vi "Read an entire module using Varaible Nodes.vi"() -> ()   [LabVIEW 2025]
panel:
  in  "stop":bool
  out "Data":dbl[](array[numeric])
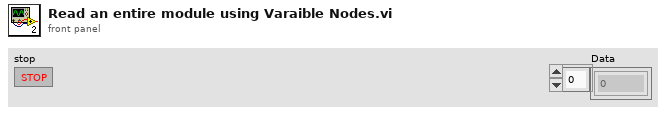
[diagram p1: front panel]
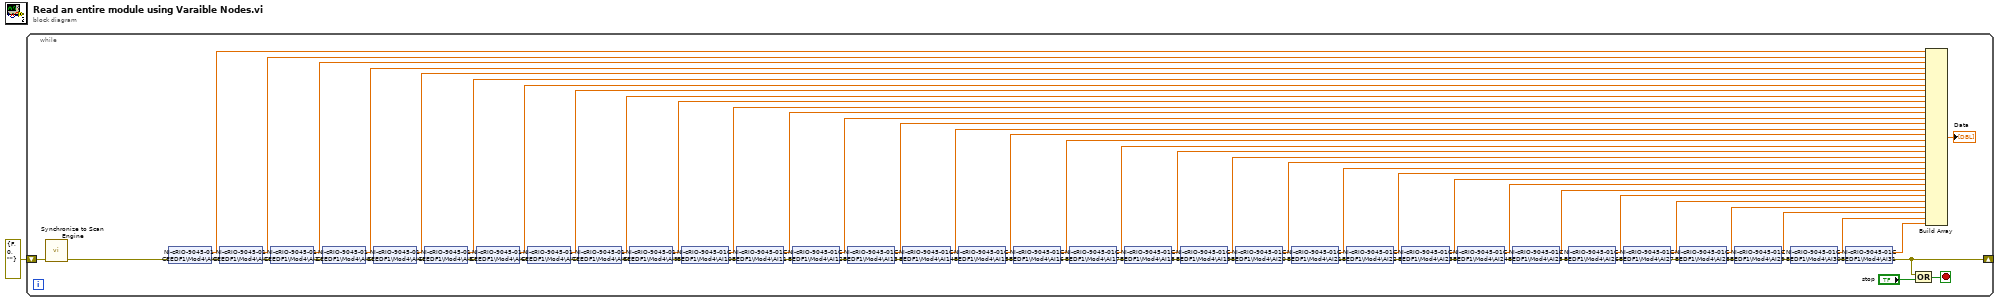
[diagram p0: block diagram]
diagram:
  n1 = while {
    shift-right: [w3] -> _
    shift-left: errorcluster {"status"=FALSE, "code"=0, "source"=""} ("error IO") -> [w2]
    stop <- w5 stop-if-true
    n2 = call <vilib>:"Synchronize to Scan Engine.vi"("error in (no error)"=w2) -> ("error out"=w4:errorcluster)  [unwired: 9 in, 1 out]
    n3 = shared-variable "NI-cRIO-9045-01CEEDF1\\Mod4\\AI0"(error in=w4) -> (w8:dbl, error out=w70:errorcluster)
    n4 = shared-variable "NI-cRIO-9045-01CEEDF1\\Mod4\\AI1"(error in=w70) -> (w9:dbl, error out=w69:errorcluster)
    n5 = shared-variable "NI-cRIO-9045-01CEEDF1\\Mod4\\AI2"(error in=w69) -> (w10:dbl, error out=w68:errorcluster)
    n6 = shared-variable "NI-cRIO-9045-01CEEDF1\\Mod4\\AI3"(error in=w68) -> (w11:dbl, error out=w67:errorcluster)
    n7 = shared-variable "NI-cRIO-9045-01CEEDF1\\Mod4\\AI4"(error in=w67) -> (w12:dbl, error out=w66:errorcluster)
    n8 = shared-variable "NI-cRIO-9045-01CEEDF1\\Mod4\\AI5"(error in=w66) -> (w13:dbl, error out=w65:errorcluster)
    n9 = shared-variable "NI-cRIO-9045-01CEEDF1\\Mod4\\AI6"(error in=w65) -> (w14:dbl, error out=w64:errorcluster)
    n10 = shared-variable "NI-cRIO-9045-01CEEDF1\\Mod4\\AI7"(error in=w64) -> (w15:dbl, error out=w63:errorcluster)
    n11 = shared-variable "NI-cRIO-9045-01CEEDF1\\Mod4\\AI8"(error in=w63) -> (w16:dbl, error out=w62:errorcluster)
    n12 = shared-variable "NI-cRIO-9045-01CEEDF1\\Mod4\\AI9"(error in=w62) -> (w17:dbl, error out=w61:errorcluster)
    n13 = shared-variable "NI-cRIO-9045-01CEEDF1\\Mod4\\AI10"(error in=w61) -> (w18:dbl, error out=w60:errorcluster)
    n14 = shared-variable "NI-cRIO-9045-01CEEDF1\\Mod4\\AI11"(error in=w60) -> (w19:dbl, error out=w59:errorcluster)
    n15 = shared-variable "NI-cRIO-9045-01CEEDF1\\Mod4\\AI12"(error in=w59) -> (w20:dbl, error out=w58:errorcluster)
    n16 = shared-variable "NI-cRIO-9045-01CEEDF1\\Mod4\\AI13"(error in=w58) -> (w21:dbl, error out=w57:errorcluster)
    n17 = shared-variable "NI-cRIO-9045-01CEEDF1\\Mod4\\AI14"(error in=w57) -> (w22:dbl, error out=w56:errorcluster)
    n18 = shared-variable "NI-cRIO-9045-01CEEDF1\\Mod4\\AI15"(error in=w56) -> (w23:dbl, error out=w55:errorcluster)
    n19 = shared-variable "NI-cRIO-9045-01CEEDF1\\Mod4\\AI16"(error in=w55) -> (w24:dbl, error out=w54:errorcluster)
    n20 = shared-variable "NI-cRIO-9045-01CEEDF1\\Mod4\\AI17"(error in=w54) -> (w25:dbl, error out=w53:errorcluster)
    n21 = shared-variable "NI-cRIO-9045-01CEEDF1\\Mod4\\AI18"(error in=w53) -> (w26:dbl, error out=w52:errorcluster)
    n22 = shared-variable "NI-cRIO-9045-01CEEDF1\\Mod4\\AI19"(error in=w52) -> (w27:dbl, error out=w51:errorcluster)
    n23 = shared-variable "NI-cRIO-9045-01CEEDF1\\Mod4\\AI20"(error in=w51) -> (w28:dbl, error out=w50:errorcluster)
    n24 = shared-variable "NI-cRIO-9045-01CEEDF1\\Mod4\\AI21"(error in=w50) -> (w29:dbl, error out=w49:errorcluster)
    n25 = shared-variable "NI-cRIO-9045-01CEEDF1\\Mod4\\AI22"(error in=w49) -> (w30:dbl, error out=w48:errorcluster)
    n26 = shared-variable "NI-cRIO-9045-01CEEDF1\\Mod4\\AI23"(error in=w48) -> (w31:dbl, error out=w47:errorcluster)
    n27 = shared-variable "NI-cRIO-9045-01CEEDF1\\Mod4\\AI24"(error in=w47) -> (w32:dbl, error out=w46:errorcluster)
    n28 = shared-variable "NI-cRIO-9045-01CEEDF1\\Mod4\\AI25"(error in=w46) -> (w33:dbl, error out=w45:errorcluster)
    n29 = shared-variable "NI-cRIO-9045-01CEEDF1\\Mod4\\AI26"(error in=w45) -> (w34:dbl, error out=w44:errorcluster)
    n30 = shared-variable "NI-cRIO-9045-01CEEDF1\\Mod4\\AI27"(error in=w44) -> (w35:dbl, error out=w43:errorcluster)
    n31 = shared-variable "NI-cRIO-9045-01CEEDF1\\Mod4\\AI28"(error in=w43) -> (w36:dbl, error out=w42:errorcluster)
    n32 = shared-variable "NI-cRIO-9045-01CEEDF1\\Mod4\\AI29"(error in=w42) -> (w37:dbl, error out=w41:errorcluster)
    n33 = shared-variable "NI-cRIO-9045-01CEEDF1\\Mod4\\AI30"(error in=w41) -> (w38:dbl, error out=w40:errorcluster)
    n34 = shared-variable "NI-cRIO-9045-01CEEDF1\\Mod4\\AI31"(error in=w40) -> (w39:dbl, error out=w3:errorcluster)
    n35 = Compound Arithmetic op=OR(w3, "stop") -> (w5:bool)
    n36 = Build Array(w8, w9, w10, w11, w12, w13, w14, w15, w16, w17, w18, w19, w20, w21, w22, w23, w24, w25, w26, w27, w28, w29, w30, w31, w32, w33, w34, w35, w36, w37, w38, w39) -> (→"Data":dbl[])
  }
